vi "Remove Char from String.vi"(2 "char to delete (0x00)":string="\u0000", 3 "string in":string="ProgramNumber=2\r\nProgramDefined=YES\r\nProgramDisabled=NO\r\nProgramName=Program 2\u0000\u0000\u0000\u0000\u0000\u0000\u0000\r\nProgramFreqTable[00]Allowed=YES\r\nProgramFreqTable[01]Allowed=YES\r\nProgramFreqTable[02]Allowed=YES\r\nProgramFreqTable[03]Allowed=YES\r\nProgramFreqTable[04]Allowed=YES\r\nProgramFreqTable[05]Allowed=YES\r\nProgramFreqTable[06]Allowed=YES\r\nProgramFreqTable[07]Allowed=YES\r\nProgramFreqTable[08]Allowed=YES\r\nProgramFreqTable[09]Allowed=YES\r\nProgramFreqTable[10]Allowed=YES\r\nProgramFreqTable[11]Allowed=YES\r\nProgramFreqTable[12]Allowed=YES\r\nProgramFreqTable[13]Allowed=YES\r\nProgramFreqTable[14]Allowed=YES\r\nProgramFreqTable[15]Allowed=YES\r\nProgramFreqTable[16]Allowed=YES\r\nProgramFreqTable[17]Allowed=YES\r\nProgramFreqTable[18]Allowed=YES\r\nProgramFreqTable[19]Allowed=YES\r\nProgramFreqTable[20]Allowed=YES\r\nProgramFreqTable[21]Allowed=YES\r\nProgramFreqTable[22]Allowed=YES\r\nProgramFreqTable[23]Allowed=YES\r\nProgramFreqTable[24]Allowed=YES\r\nProgramFreqTable[25]Allowed=YES\r\nProgramFreqTable[26]Allowed=YES\r\nProgramFreqTable[27]Allowed=YES\r\nProgramFreqTable[28]Allowed=YES\r\nProgramFreqTable[29]Allowed=YES\r\nProgramFreqTable[30]Allowed=YES\r\nProgramFreqTable[31]Allowed=YES\r\nProgramFreqTable[32]Allowed=YES\r\nProgramFreqTable[33]Allowed=YES\r\nProgramFreqTable[34]Allowed=YES\r\nProgramFreqTable[35]Allowed=YES\r\nProgramFreqTable[36]Allowed=YES\r\nProgramFreqTable[37]Allowed=YES\r\nProgramFreqTable[38]Allowed=YES\r\nProgramFreqTable[39]Allowed=YES\r\nProgramFreqTable[40]Allowed=YES\r\nProgramFreqTable[41]Allowed=YES\r\nProgramFreqTable[42]Allowed=YES\r\nProgramFreqTable[43]Allowed=YES\r\nProgramFreqTable[44]Allowed=YES\r\nProgramFreqTable[45]Allowed=YES\r\nProgramFreqTable[46]Allowed=YES\r\nProgramFreqTable[47]Allowed=YES\r\nProgramFreqTable[48]Allowed=YES\r\nProgramFreqTable[49]Allowed=YES\r\nProgramFreqTable[50]Allowed=YES\r\nProgramFreqTable[51]Allowed=YES\r\nProgramFreqTable[52]Allowed=YES\r\nProgramFreqTable[53]Allowed=YES\r\nProgramFreqTable[54]Allowed=YES\r\nProgramFreqTable[55]Allowed=YES\r\nProgramFreqTable[56]Allowed=YES\r\nProgramFreqTable[57]Allowed=YES\r\nProgramFreqTable[58]Allowed=YES\r\nProgramFreqTable[59]Allowed=YES\r\nProgramFreqTable[60]Allowed=YES\r\nProgramFreqTable[61]Allowed=YES\r\nProgramFreqTable[62]Allowed=YES\r\nProgramFreqTable[63]Allowed=YES\r\nProgramFrequencyIndex=0\r\nPA_Defined=YES\r\nPB_Defined=YES\r\nPC_Defined=YES\r\nPD_Defined=YES\r\n\r\n-- PULSE PA --\r\nPulseNamePA=P1\u0000\u0000\u0000\u0000\u0000\u0000\u0000\u0000\u0000\u0000\u0000\u0000\u0000\u0000\r\nAmplitudeLowLimitPA=15\r\nAmplitudeStepPA=15\r\nAmplitudeStepIndexPA=1\r\nPulseWidthLowLimitPA=10\r\nPulseWidthHighLimitPA=20\r\nPulseWidthPA=10\r\nElectrodeAmpPercentPA[CH01]=0\r\nElectrodeAmpPercentPA[CH02]=0\r\nElectrodeAmpPercentPA[CH03]=0\r\nElectrodeAmpPercentPA[CH04]=0\r\nElectrodeAmpPercentPA[CH05]=0\r\nElectrodeAmpPercentPA[CH06]=0\r\nElectrodeAmpPercentPA[CH07]=0\r\nElectrodeAmpPercentPA[CH08]=0\r\nElectrodeAmpPercentPA[CH09]=0\r\nElectrodeAmpPercentPA[CH10]=0\r\nElectrodeAmpPercentPA[CH11]=0\r\nElectrodeAmpPercentPA[CH12]=0\r\nElectrodeAmpPercentPA[CH13]=0\r\nElectrodeAmpPercentPA[CH14]=0\r\nElectrodeAmpPercentPA[CH15]=0\r\nElectrodeAmpPercentPA[CH16]=0\r\nElectrodeAmpPercentPA[CH17]=0\r\nElectrodeAmpPercentPA[CH18]=0\r\nElectrodeAmpPercentPA[CH19]=0\r\nElectrodeAmpPercentPA[CH20]=0\r\nElectrodeAmpPercentPA[CH21]=0\r\nElectrodeAmpPercentPA[CH22]=0\r\nElectrodeAmpPercentPA[CH23]=0\r\nElectrodeAmpPercentPA[CH24]=0\r\nElectrodeAmpPercentPA[CH25]=-100\r\nElectrodeAmpPercentPA[CH26]=100\r\n\r\n-- PULSE PB --\r\nPulseNamePB=P2\u0000\u0000\u0000\u0000\u0000\u0000\u0000\u0000\u0000\u0000\u0000\u0000\u0000\u0000\r\nAmplitudeLowLimitPB=15\r\nAmplitudeStepPB=15\r\nAmplitudeStepIndexPB=1\r\nPulseWidthLowLimitPB=10\r\nPulseWidthHighLimitPB=20\r\nPulseWidthPB=10\r\nElectrodeAmpPercentPB[CH01]=0\r\nElectrodeAmpPercentPB[CH02]=0\r\nElectrodeAmpPercentPB[CH03]=0\r\nElectrodeAmpPercentPB[CH04]=0\r\nElectrodeAmpPercentPB[CH05]=0\r\nElectrodeAmpPercentPB[CH06]=0\r\nElectrodeAmpPercentPB[CH07]=0\r\nElectrodeAmpPercentPB[CH08]=0\r\nElectrodeAmpPercentPB[CH09]=0\r\nElectrodeAmpPercentPB[CH10]=0\r\nElectrodeAmpPercentPB[CH11]=0\r\nElectrodeAmpPercentPB[CH12]=0\r\nElectrodeAmpPercentPB[CH13]=0\r\nElectrodeAmpPercentPB[CH14]=0\r\nElectrodeAmpPercentPB[CH15]=0\r\nElectrodeAmpPercentPB[CH16]=0\r\nElectrodeAmpPercentPB[CH17]=0\r\nElectrodeAmpPercentPB[CH18]=0\r\nElectrodeAmpPercentPB[CH19]=0\r\nElectrodeAmpPercentPB[CH20]=0\r\nElectrodeAmpPercentPB[CH21]=0\r\nElectrodeAmpPercentPB[CH22]=0\r\nElectrodeAmpPercentPB[CH23]=0\r\nElectrodeAmpPercentPB[CH24]=0\r\nElectrodeAmpPercentPB[CH25]=-100\r\nElectrodeAmpPercentPB[CH26]=100\r\n\r\n-- PULSE PC --\r\nPulseNamePC=P3\u0000\u0000\u0000\u0000\u0000\u0000\u0000\u0000\u0000\u0000\u0000\u0000\u0000\u0000\r\nAmplitudeLowLimitPC=15\r\nAmplitudeStepPC=15\r\nAmplitudeStepIndexPC=1\r\nPulseWidthLowLimitPC=10\r\nPulseWidthHighLimitPC=20\r\nPulseWidthPC=10\r\nElectrodeAmpPercentPC[CH01]=0\r\nElectrodeAmpPercentPC[CH02]=0\r\nElectrodeAmpPercentPC[CH03]=0\r\nElectrodeAmpPercentPC[CH04]=0\r\nElectrodeAmpPercentPC[CH05]=0\r\nElectrodeAmpPercentPC[CH06]=0\r\nElectrodeAmpPercentPC[CH07]=0\r\nElectrodeAmpPercentPC[CH08]=0\r\nElectrodeAmpPercentPC[CH09]=0\r\nElectrodeAmpPercentPC[CH10]=0\r\nElectrodeAmpPercentPC[CH11]=0\r\nElectrodeAmpPercentPC[CH12]=0\r\nElectrodeAmpPercentPC[CH13]=0\r\nElectrodeAmpPercentPC[CH14]=0\r\nElectrodeAmpPercentPC[CH15]=0\r\nElectrodeAmpPercentPC[CH16]=0\r\nElectrodeAmpPercentPC[CH17]=0\r\nElectrodeAmpPercentPC[CH18]=0\r\nElectrodeAmpPercentPC[CH19]=0\r\nElectrodeAmpPercentPC[CH20]=0\r\nElectrodeAmpPercentPC[CH21]=0\r\nElectrodeAmpPercentPC[CH22]=0\r\nElectrodeAmpPercentPC[CH23]=0\r\nElectrodeAmpPercentPC[CH24]=0\r\nElectrodeAmpPercentPC[CH25]=-100\r\nElectrodeAmpPercentPC[CH26]=100\r\n\r\n-- PULSE PD --\r\nPulseNamePD=P4\u0000\u0000\u0000\u0000\u0000\u0000\u0000\u0000\u0000\u0000\u0000\u0000\u0000\u0000\r\nAmplitudeLowLimitPD=15\r\nAmplitudeStepPD=15\r\nAmplitudeStepIndexPD=1\r\nPulseWidthLowLimitPD=10\r\nPulseWidthHighLimitPD=20\r\nPulseWidthPD=10\r\nElectrodeAmpPercentPD[CH01]=0\r\nElectrodeAmpPercentPD[CH02]=0\r\nElectrodeAmpPercentPD[CH03]=0\r\nElectrodeAmpPercentPD[CH04]=0\r\nElectrodeAmpPercentPD[CH05]=0\r\nElectrodeAmpPercentPD[CH06]=0\r\nElectrodeAmpPercentPD[CH07]=0\r\nElectrodeAmpPercentPD[CH08]=0\r\nElectrodeAmpPercentPD[CH09]=0\r\nElectrodeAmpPercentPD[CH10]=0\r\nElectrodeAmpPercentPD[CH11]=0\r\nElectrodeAmpPercentPD[CH12]=0\r\nElectrodeAmpPercentPD[CH13]=0\r\nElectrodeAmpPercentPD[CH14]=0\r\nElectrodeAmpPercentPD[CH15]=0\r\nElectrodeAmpPercentPD[CH16]=0\r\nElectrodeAmpPercentPD[CH17]=0\r\nElectrodeAmpPercentPD[CH18]=0\r\nElectrodeAmpPercentPD[CH19]=0\r\nElectrodeAmpPercentPD[CH20]=0\r\nElectrodeAmpPercentPD[CH21]=0\r\nElectrodeAmpPercentPD[CH22]=0\r\nElectrodeAmpPercentPD[CH23]=0\r\nElectrodeAmpPercentPD[CH24]=0\r\nElectrodeAmpPercentPD[CH25]=-100\r\nElectrodeAmpPercentPD[CH26]=100") -> (0 "deleted count":i32=-1, 1 "string out":string)   [LabVIEW 2010]
doc: "This function deletes all occurrences of a single character in a string. It is particularly useful for deleting nul bytes (0x00) that can be present in the middle of a LabView string."
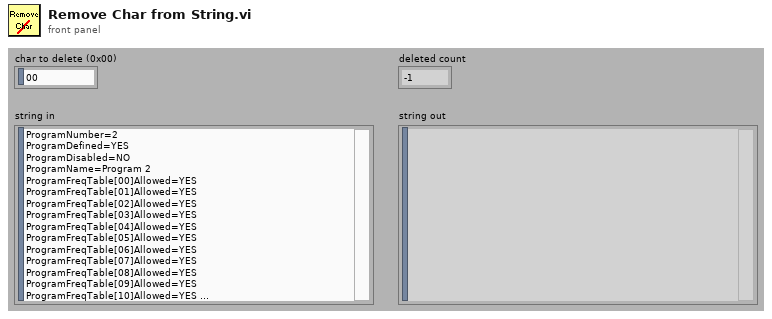
[diagram p1: front panel]
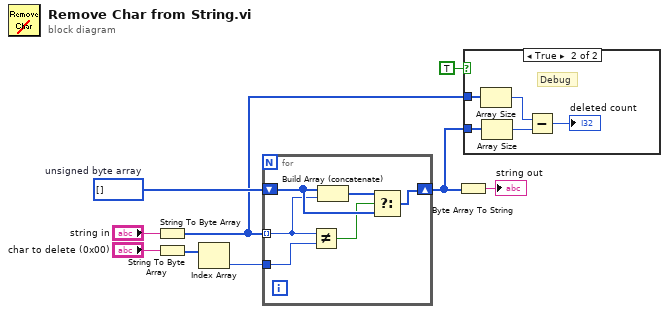
[diagram p0: block diagram]
diagram:
  w7 = u8[] []  # unsigned byte array
  n1 = String To Byte Array(string="string in") -> (unsigned byte array=w3:u8[])
  n2 = String To Byte Array(string="char to delete (0x00)") -> (unsigned byte array=w6:u8[])
  n3 = Index Array(array=w6) -> (element=w4:u8)  [unwired: 1 in]
  n4 = for {
    shift-right: [w15] -> w2
    shift-left: w7 -> [w13]
    tunnel: w3 -> [w12] mode=indexing
    tunnel: w4 -> [w11]
    n5 = Not Equal?(x=w12, y=w11) -> (x != y?=w10:bool)
    n6 = Build Array (concatenate)(w13, w12) -> (w14:u8[])
    n7 = Select(t=w14, s=w10, f=w13) -> (s? t:f=w15:u8[])
  }
  n8 = Byte Array To String(unsigned byte array=w2) -> (string=→"string out":string)
  n9 = case shown="True" TRUE {
    tunnel: w3 -> [_ w20]
    tunnel: w2 -> [_ w19]
    frame False {
    }
    frame True {
      # "Debug"
      n10 = Array Size(array=w20) -> (size(s)=w18:i32)
      n11 = Array Size(array=w19) -> (size(s)=w17:i32)
      n12 = Subtract(x=w18, y=w17) -> (x-y=→"deleted count":i32)
    }
  }
